vi "jettl Msg Setup.vi"() -> (2 "Msg Strategy":refnum<class "Msg Strategy.lvclass">)   [LabVIEW 2021, in "Setup Msg Strategy.lvlib"]
uses:
  Setup Msg Strategy.lvlib
  Setup Msg Strategy/Setup Msg Strategy.lvclass
  C:/git/jettl/jettl/jettl Msg Setup/Setup Msg Strategy/Setup Msg Strategy.lvclass
  C:/git/jettl/jettl/jettl/Msg Strategy/Msg Strategy.lvclass
  jettl/Msg Strategy/Msg Strategy.lvclass
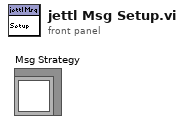
[diagram p1: front panel]
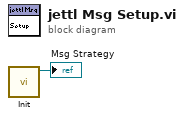
[diagram p0: block diagram]
diagram:
  n1 = call "Init.vi"() -> ("Setup Msg Strategy out"=→"Msg Strategy":refnum<class "Setup Msg Strategy.lvclass">)  [unwired: 11 in]
